vi "Test_WriteValue_CheckTerminal_TerminalUpdated.vi"(8 "error in (no error)":errorcluster, 11 "TestCase in":refnum<class "TestFormattedStringBinding.lvclass">) -> (0 "error out":errorcluster, 3 "TestCase out":refnum<class "TestFormattedStringBinding.lvclass">)   [LabVIEW 2017, in "TestFormattedStringBinding.lvclass"]
uses:
  TestFormattedStringBinding.lvclass
  Source/Concrete/FormattedStringBinding/FormattedStringBinding.lvclass/FormattedStringBinding.ctl
  Source/Concrete/FormattedStringBinding/FormattedStringBinding.lvclass
  C:/Git/composed-transport/Source/Concrete/TerminalValueBinding/TerminalValueBinding.lvclass
  C:/Git/composed-transport/Source/ITransport/ITransport.lvclass
  <vilib>/Utility/error.llb/Error Cluster From Error Code.vi
  Source/Concrete/TerminalValueBinding/Construct Terminal Value Binding.vi
  Source/ITransport/ITransport.lvclass
panel:
  in  "String":string
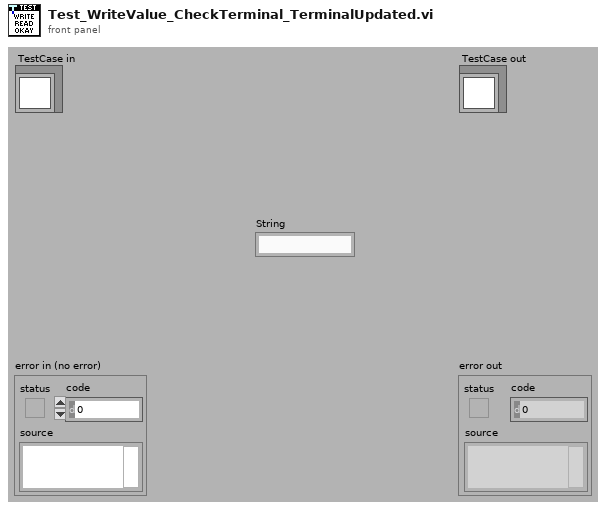
[diagram p1: front panel]
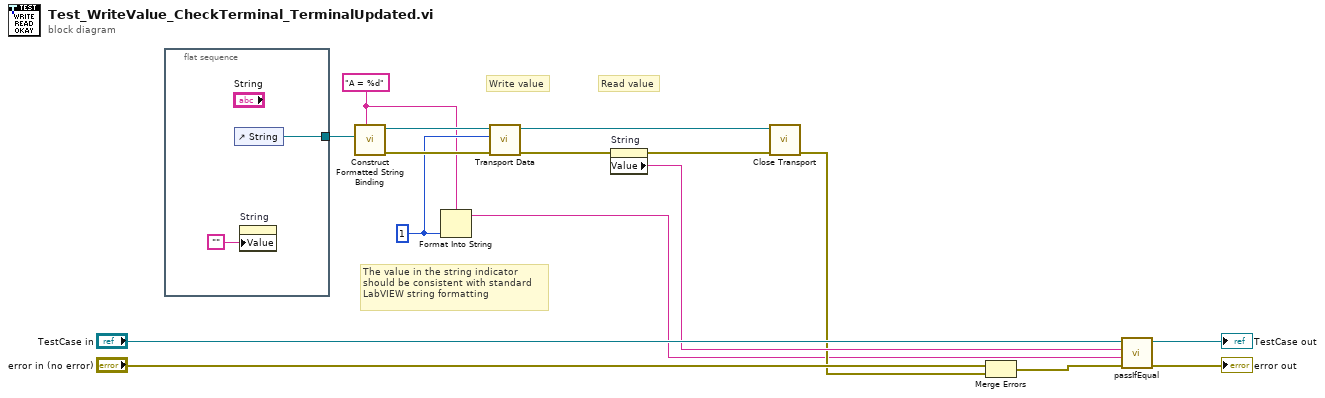
[diagram p0: block diagram]
diagram:
  w2 = "A = %d" ("Format String")
  w3 = 1
  # "The value in the string indicator\nshould be consistent with standard\nLabVIEW string formatting"
  # "Read value"
  # "Write value"
  n1 = flat-sequence {
    tunnel: [w18] -> w8
    frame #0 {
      n2 = control-ref of="String"() -> (w18:refnum<vi>)
      n3 = property on="String" class="Str"("Value"="") -> ()  [unwired: 2 in, 2 out]
    }
  }
  n4 = call "Construct Formatted String Binding.vi"("Format String"=w2, "Str Refnum"=w8) -> ("error out"=w10:errorcluster, "FormattedStringBinding"=w12:refnum<class "FormattedStringBinding.lvclass">)  [unwired: 8 in]
  n5 = Format Into String(format string=w2, w3) -> (resulting string=w1:string)  [unwired: 2 in, 1 out]
  n6 = call "Transport Data.vi"("error in (no error)"=w10, "Value"=w3, "ITransport in"=w12) -> ("error out"=w7:errorcluster, "ITransport out"=w9:refnum<class "FormattedStringBinding.lvclass">)  [unwired: 7 in]
  n7 = property on="String" class="Str"(error in=w7) -> (error out=w6:errorcluster, "Value"=w5:string)  [unwired: 1 in, 1 out]
  n8 = call-dynamic "Close Transport.vi"("error in (no error)"=w6, "ITransport in"=w9) -> ("error out"=w4:errorcluster)  [unwired: 9 in]
  n9 = Merge Errors("error in (no error)", w4) -> (w11:errorcluster)
  n10 = call-dynamic "passIfEqual.vi"("error in (no error)"=w11, "y"=w1, "x"=w5, "TestCase in"="TestCase in") -> ("error out"=→"error out":errorcluster, "TestCase out"=→"TestCase out":refnum<class "TestFormattedStringBinding.lvclass">)  [unwired: 6 in]
